vi "FlatSequence.vi"() -> ()   [LabVIEW 2020]
panel:
  out "Tank 3":dbl(slide) scale=0.0..100.0
  out "Tank 2":dbl(slide) scale=0.0..100.0
  out "Tank":dbl(slide) scale=0.0..100.0
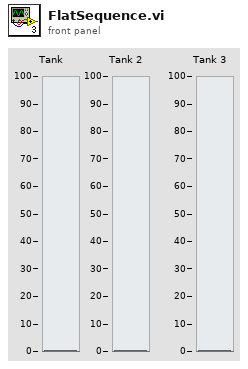
[diagram p1: front panel]
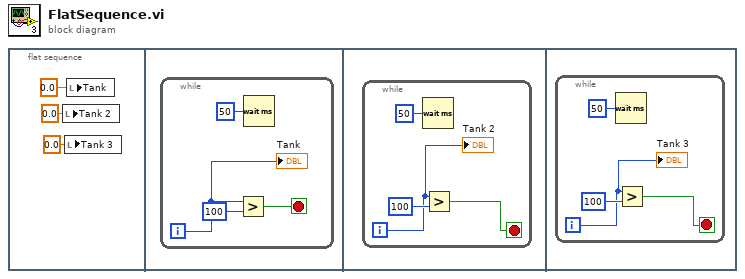
[diagram p0: block diagram]
diagram:
  n1 = flat-sequence {
    frame #0 {
      n2 = local write "Tank 2"(0.0 ("Tank")) -> ()
      n3 = local write "Tank 3"(0.0 ("Tank")) -> ()
      n4 = local write "Tank"(0.0 ("Tank")) -> ()
    }
    frame #1 {
      n5 = while {
        i -> [w7]
        stop <- w5 stop-if-true
        n6 = Greater?(x=w7, y=100) -> (0:w5:bool)
        n7 = Wait (ms)(milliseconds to wait=u32 50) -> ()  [unwired: 1 out]
        "Tank" <- w7
      }
    }
    frame #2 {
      n8 = while {
        i -> [w10]
        stop <- w9 stop-if-true
        n9 = Wait (ms)(milliseconds to wait=u32 50) -> ()  [unwired: 1 out]
        n10 = Greater?(x=w10, y=100) -> (0:w9:bool)
        "Tank 2" <- w10
      }
    }
    frame #3 {
      n11 = while {
        i -> [w12]
        stop <- w14 stop-if-true
        n12 = Wait (ms)(milliseconds to wait=u32 50) -> ()  [unwired: 1 out]
        n13 = Greater?(x=w12, y=100) -> (0:w14:bool)
        "Tank 3" <- w12
      }
    }
  }
